vi "PH_Beckhoff-16BB_Testtool.ProcEvents.vi"(0 "i ref in":refnum<vi>, 5 "error in (no error)":errorcluster) -> (14 "i ref out":refnum<vi>, 19 "error out":errorcluster)   [LabVIEW 2014, in "PH_Beckhoff-16BB_Testtool.lvlib"]
doc: "This method is used to define the events the object will listen to. Add your own events here."
uses:
  PH_Beckhoff-16BB_Testtool.lvlib
  CS_Core/BaseProcess/BaseProcess.lvlib
  PH_Basics/PH_Common/PH_Common.lvlib
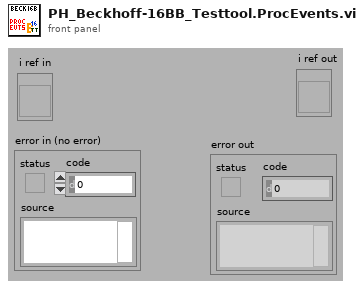
[diagram p1: front panel]
types:
  T1 = typedef "PH_Beckhoff-16BB_Testtool.lvlib/PH_Beckhoff-16BB_Testtool.i attribute.ctl" = cluster{"GUI Refs":refnum<vi>[], "16BB Instance":string}
  T2 = typedef "PH_Common.lvlib/PH_DIM.Event Declarer.ctl" = cluster{"Service Name":string, "Selector":string}
  T3 = typedef "BaseProcess.lvlib/BaseProcess.event definition.ctl" = cluster{"CAEEvtDef":T4, "Data Descriptor":T5}
  T4 = typedef "CAEObj.lvlib/CAEObj.event definition.ctl" = cluster{"URL":string, "enable":bool, "ignoreResID":bool}
  T5 = typedef "BaseProcess.lvlib/BaseProcess.descriptor string definition.ctl" = string
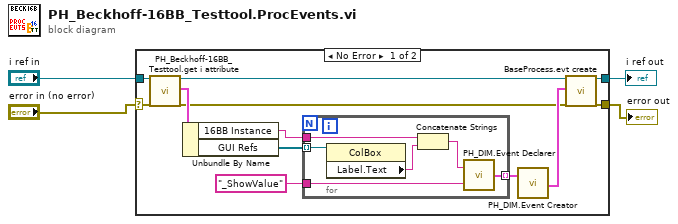
[diagram p0: block diagram]
diagram:
  n1 = case shown="No Error" "error in (no error)" {
    selector: "error in (no error)" -> [w13 w23]
    tunnel: "i ref in" -> [w11 w24]
    tunnel: [w16 w23] -> w3
    tunnel: [w15 w24] -> w2
    frame No Error {
      n2 = call "PH_Beckhoff-16BB_Testtool.get i attribute.vi"("i ref in"=w11, "error in (no error)"=w13) -> ("i ref out"=w6:refnum<vi>, "i attribute"=w10:T1, "error out"=w5:errorcluster)  [unwired: 15 in]
      n3 = Unbundle By Name(w10) -> ("16BB Instance"=w7:string, "GUI Refs"=w9:refnum<vi>[])
      n4 = for {
        tunnel: [w22] -> w14 mode=indexing
        tunnel: "_ShowValue" -> [w21]
        tunnel: w7 -> [w20]
        tunnel: w9 -> [w19] mode=indexing
        n5 = property class="ColBox"(reference=w19) -> ("Label.Text"=w18:string)  [unwired: 1 in, 2 out]
        n6 = Concatenate Strings(w20, w18) -> (w17:string)
        n7 = call "PH_DIM.Event Declarer.vi"("Selector"=w21, "Service Name"=w17) -> ("declared DIM Event"=w22:T2)
      }
      n8 = call "PH_DIM.Event Creator.vi"("Trendmessage Services"=w14) -> ("DIM Service Events"=w8:T3[])  [unwired: 18 in]
      n9 = call "BaseProcess.evt create.vi"("i ref in"=w6, "newEvents"=w8, "error in (no error)"=w5) -> ("i ref out"=w15:refnum<vi>, "error out"=w16:errorcluster)  [unwired: 13 in, 2 out]
    }
    frame Error {
    }
  }
  "i ref out" <- w2
  "error out" <- w3
